vi "Load Selected Device Info.vi"(8 "error in":errorcluster, 11 "Selected Device":string) -> (0 "error out":errorcluster)   [LabVIEW 2024, in "Data Base.lvlib"]
uses:
  Data Base.lvlib
  Support/General Type Defs/Device Data.ctl
  Support/General Type Defs/Device OS.ctl
  Support/General Type Defs/Global Data.vi
  Support/General Type Defs/General Type Definitions.lvlib
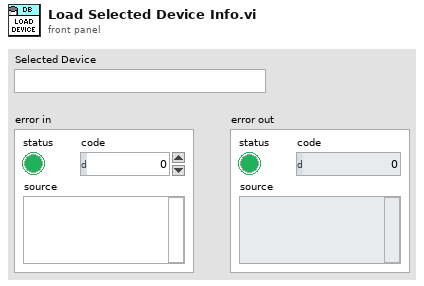
[diagram p1: front panel]
types:
  T1 = typedef "General Type Definitions.lvlib/Device Data.ctl" = cluster{"OS":T2, "User":string, "Password":string, "Hostname":string, "IP Address":string}
  T2 = typedef "General Type Definitions.lvlib/Device OS.ctl" = enum16{"Windows", "Linux"}
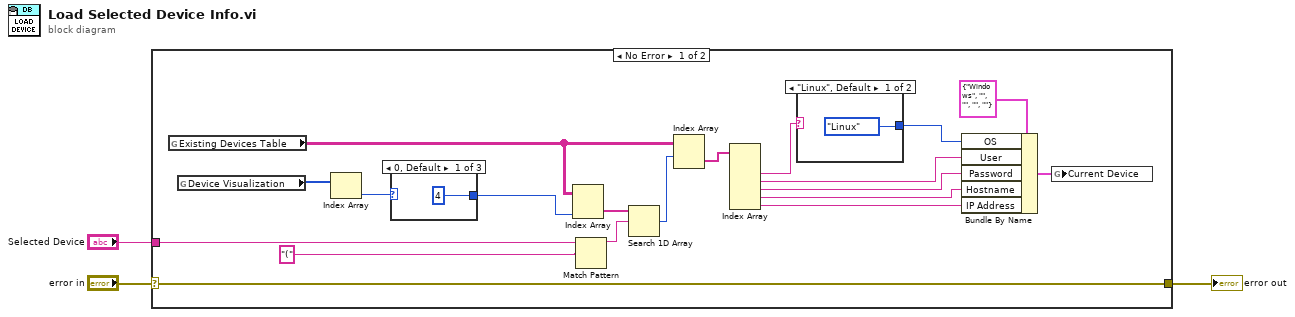
[diagram p0: block diagram]
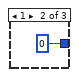
[diagram p2: hidden frame]
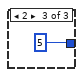
[diagram p3: hidden frame]
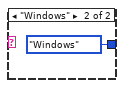
[diagram p4: hidden frame]
diagram:
  n1 = case shown="No Error" "error in" {
    selector: "error in" -> [w10 w28]
    tunnel: "Selected Device" -> [w9 _]
    tunnel: [w10 w28] -> w1
    frame No Error {
      n2 = global read "Global Data.vi" "Existing Devices Table"() -> (w20:string[][])
      n3 = global read "Global Data.vi" "Device Visualization"() -> (w6:i32[])
      n4 = Index Array(array=w6) -> (element=w5:i32)  [unwired: 1 in]
      n5 = case shown="0, Default" w5 {
        tunnel: [4 ("index (col)") 0 ("index (col)") 5 ("index (col)")] -> w4
        frame 0, Default {
        }
        frame 1 {
        }
        frame 2 {
        }
      }
      n6 = Index Array(array=w20, index (col)=w4) -> (element=w22:string[])  [unwired: 1 in]
      n7 = Match Pattern(string=w9, regular expression="(") -> (before substring=w7:string)  [unwired: 1 in, 3 out]
      n8 = Search 1D Array(1D array=w22, element=w7) -> (index of element=w19:i32)  [unwired: 1 in]
      n9 = Index Array(array=w20, index (row)=w19) -> (element=w18:string[])  [unwired: 1 in]
      n10 = Index Array(array=w18) -> (element #2=w12:string, element #3=w13:string, element #4=w17:string, element #5=w16:string, element #6=w15:string)  [unwired: 6 in, 1 out]
      n11 = case shown="\"Linux\", Default" w12 {
        tunnel: [Device_OS."Linux" ("OS") Device_OS."Windows" ("OS")] -> w11
        frame "Linux", Default {
        }
        frame "Windows" {
        }
      }
      n12 = Bundle By Name(cluster=T1 {"OS"=enum."Windows", "User"="", "Password"="", "Hostname"="", "IP Address"=""} ("Device Data"), "OS"=w11, "User"=w13, "Password"=w17, "Hostname"=w16, "IP Address"=w15) -> (w14:T1)
      n13 = global write "Global Data.vi" "Current Device"(w14) -> ()
    }
    frame Error {
    }
  }
  "error out" <- w1
